vi "Attach Param - Decimal.vi"(8 "Error in":errorcluster caption="Error in (no error)", 9 "Value":i32, 10 "Param Name":string, 11 "Params Array In":T1[](array[typedef])) -> (0 "Error out":errorcluster, 3 "Params Array Out":T1[](array[typedef])=[{"Param"="user_field_names", "Value"="0"}])   [LabVIEW 2018]
uses:
  TypeDef/Param.ctl
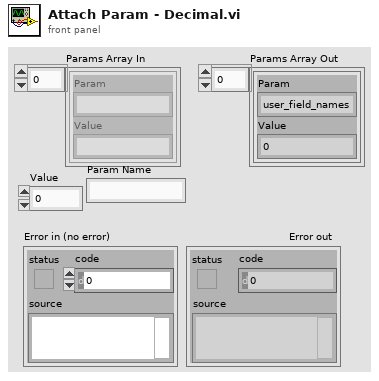
[diagram p1: front panel]
types:
  T1 = typedef "Param.ctl" = cluster{"Param":string, "Value":string}
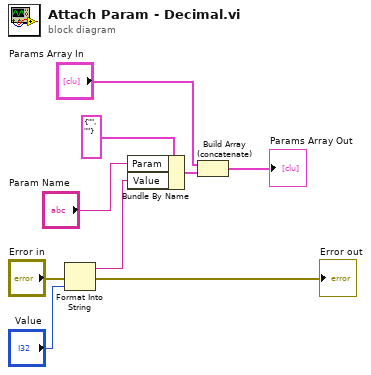
[diagram p0: block diagram]
diagram:
  n1 = Format Into String(error in="Error in", "Value") -> (resulting string=w1:string, error out=→"Error out":errorcluster)  [unwired: 2 in]
  n2 = Bundle By Name(cluster=T1 {"Param"="", "Value"=""} ("Cluster"), "Param"="Param Name", "Value"=w1) -> (w6:T1)
  n3 = Build Array (concatenate)("Params Array In", w6) -> (→"Params Array Out":T1[])
